vi "Main.vi"(8 "error in (no error)":errorcluster, 11 "AOTFBase in":refnum<class "AOTF.lvclass">) -> (0 "error out":errorcluster, 3 "component":refnum<class "AOTF.lvclass">)   [LabVIEW 2012, in "AOTF.lvclass"]
doc: "Main VI of the component."
uses:
  AOTF.lvclass
  <vilib>/Distrio/Murmex/Murmex/command_enum.ctl
  Controls/laser line ring.ctl
  <vilib>/Distrio/Murmex/InitialiseMessage/InitialiseMessage.lvclass
  AOTF.lvclass/AOTF.ctl
  <vilib>/Distrio/Murmex/ConfigureMessage/ConfigureMessage.lvclass
  <vilib>/Distrio/Murmex/TerminateMessage/TerminateMessage.lvclass
  <vilib>/Distrio/Murmex/Murmex/update_cluster.ctl
  <vilib>/Distrio/Murmex/Murmex/Set configure at initialise.vi
  <vilib>/Distrio/Murmex/Murmex/Set VI reference.vi
  <vilib>/Distrio/Murmex/Murmex/Get ID.vi
  <vilib>/Distrio/Murmex/Murmex/Set log reference.vi
  <vilib>/Distrio/Murmex/Murmex/Set write log to disk.vi
  <vilib>/Distrio/Murmex/Murmex/Murmex.lvclass
  <vilib>/Distrio/Murmex/Message/Message.lvclass
panel:
  in  "button::configure":bool
  in  "button::quit":bool
  out "terminate?":bool=TRUE
  in  "Tab Control":enum32{"Main", "Ramp", "Debug"}(tab)
  in  "Power":dbl(knob) caption="Power [%]" min=0.0 max=100.0 scale=0.0..100.0
  in  "Wavelength":T1=10 items=["Blind"=10, "405nm"=0, "445nm"=5, "491nm"=1, "515nm"=2, "561nm"=3]
  in  "Frame rate (Hz)":dbl
  in  "Number of frames":i32
  in  "Final power [%]":dbl
  in  "Start power [%]":dbl
  out "log":string="\r\n11:11:41.970 05/12/2013: initialise from AOTF to AOTF\r\n11:11:42.586 05/12/2013: inform from AOTF to AOTF\r\n11:11:43.913 05/12/2013: update from AOTF to AOTF\r\n11:11:45.142 05/12/2013: generic (shutter_off) from AOTF to AOTF\r\n11:11:45.270 05/12/2013: generic (shutter_on) from AOTF to AOTF\r\n11:11:45.902 05/12/2013: generic (shutter_off) from AOTF to AOTF\r\n11:11:45.932 05/12/2013: inspect from AOTF to AOTF\r\n11:11:48.013 05/12/2013: configure from AOTF to AOTF\r\n11:11:52.003 05/12/2013: inform from AOTF to AOTF\r\n11:11:58.521 05/12/2013: initialise from AOTF to AOTF\r\n11:11:58.561 05/12/2013: inform from AOTF to AOTF\r\n11:11:58.695 05/12/2013: inform from AOTF to AOTF\r\n11:12:02.089 05/12/2013: update from AOTF to AOTF\r\n11:12:02.308 05/12/2013: inspect from AOTF to AOTF\r\n11:12:02.364 05/12/2013: inform from AOTF to AOTF\r\n11:12:05.062 05/12/2013: generic (shutter_on) from AOTF to AOTF\r\n11:12:06.690 05/12/2013: update from AOTF to AOTF\r\n11:12:06.909 05/12/2013: inspect from AOTF to AOTF\r\n11:12:06.964 05/12/2013: inform from AOTF to AOTF\r\n11:12:07.770 05/12/2013: update from AOTF to AOTF\r\n11:12:07.989 05/12/2013: inspect from AOTF to AOTF\r\n11:12:08.044 05/12/2013: inform from AOTF to AOTF\r\n11:12:08.627 05/12/2013: update from AOTF to AOTF\r\n11:12:08.846 05/12/2013: inspect from AOTF to AOTF\r\n11:12:08.900 05/12/2013: inform from AOTF to AOTF\r\n11:12:09.290 05/12/2013: update from AOTF to AOTF\r\n11:12:09.508 05/12/2013: inspect from AOTF to AOTF\r\n11:12:09.563 05/12/2013: inform from AOTF to AOTF\r\n11:12:10.154 05/12/2013: update from AOTF to AOTF\r\n11:12:10.373 05/12/2013: inspect from AOTF to AOTF\r\n11:12:10.430 05/12/2013: inform from AOTF to AOTF\r\n11:12:20.953 05/12/2013: update from AOTF to AOTF\r\n11:12:21.172 05/12/2013: inspect from AOTF to AOTF\r\n11:12:21.227 05/12/2013: inform from AOTF to AOTF\r\n11:12:22.057 05/12/2013: update from AOTF to AOTF\r\n11:12:22.276 05/12/2013: inspect from AOTF to AOTF\r\n11:12:22.330 05/12/2013: inform from AOTF to AOTF\r\n11:12:22.841 05/12/2013: update from AOTF to AOTF\r\n11:12:23.060 05/12/2013: inspect from AOTF to AOTF\r\n11:12:23.114 05/12/2013: inform from AOTF to AOTF\r\n11:12:23.449 05/12/2013: update from AOTF to AOTF\r\n11:12:23.668 05/12/2013: inspect from AOTF to AOTF\r\n11:12:23.724 05/12/2013: inform from AOTF to AOTF\r\n11:12:24.514 05/12/2013: update from AOTF to AOTF\r\n11:12:24.733 05/12/2013: inspect from AOTF to AOTF\r\n11:12:24.789 05/12/2013: inform from AOTF to AOTF\r\n11:12:25.098 05/12/2013: update from AOTF to AOTF\r\n11:12:25.317 05/12/2013: inspect from AOTF to AOTF\r\n11:12:25.371 05/12/2013: inform from AOTF to AOTF\r\n11:12:26.482 05/12/2013: update from AOTF to AOTF\r\n11:12:26.701 05/12/2013: inspect from AOTF to AOTF\r\n11:12:26.755 05/12/2013: inform from AOTF to AOTF\r\n11:12:27.154 05/12/2013: update from AOTF to AOTF\r\n11:12:27.373 05/12/2013: inspect from AOTF to AOTF\r\n11:12:27.428 05/12/2013: inform from AOTF to AOTF\r\n11:12:27.666 05/12/2013: update from AOTF to AOTF\r\n11:12:27.885 05/12/2013: inspect from AOTF to AOTF\r\n11:12:27.944 05/12/2013: inform from AOTF to AOTF\r\n11:12:33.380 05/12/2013: update from AOTF to AOTF\r\n11:12:33.484 05/12/2013: update from AOTF to AOTF\r\n11:12:33.603 05/12/2013: inspect from AOTF to AOTF\r\n11:12:33.611 05/12/2013: update from AOTF to AOTF\r\n11:12:33.684 05/12/2013: update from AOTF to AOTF\r\n11:12:33.740 05/12/2013: update from AOTF to AOTF\r\n11:12:33.827 05/12/2013: inspect from AOTF to AOTF\r\n11:12:33.835 05/12/2013: update from AOTF to AOTF\r\n11:12:33.897 05/12/2013: inform from AOTF to AOTF\r\n11:12:33.903 05/12/2013: update from AOTF to AOTF\r\n11:12:33.940 05/12/2013: update from AOTF to AOTF\r\n11:12:34.085 05/12/2013: update from AOTF to AOTF\r\n11:12:34.119 05/12/2013: inspect from AOTF to AOTF\r\n11:12:34.292 05/12/2013: update from AOTF to AOTF\r\n11:12:34.336 05/12/2013: inspect from AOTF to AOTF\r\n11:12:34.553 05/12/2013: inspect from AOTF to AOTF\r\n11:12:34.608 05/12/2013: inform from AOTF to AOTF\r\n11:12:34.739 05/12/2013: update from AOTF to AOTF\r\n11:12:34.771 05/12/2013: update from AOTF to AOTF\r\n11:12:34.826 05/12/2013: inspect from AOTF to AOTF\r\n11:12:34.834 05/12/2013: update from AOTF to AOTF\r\n11:12:34.867 05/12/2013: update from AOTF to AOTF\r\n11:12:34.931 05/12/2013: update from AOTF to AOTF\r\n11:12:34.979 05/12/2013: update from AOTF to AOTF\r\n11:12:35.003 05/12/2013: update from AOTF to AOTF\r\n11:12:35.027 05/12/2013: update from AOTF to AOTF\r\n11:12:35.041 05/12/2013: update from AOTF to AOTF\r\n11:12:35.051 05/12/2013: inspect from AOTF to AOTF\r\n11:12:35.066 05/12/2013: update from AOTF to AOTF\r\n11:12:35.116 05/12/2013: update from AOTF to AOTF\r\n11:12:35.171 05/12/2013: update from AOTF to AOTF\r\n11:12:35.211 05/12/2013: update from AOTF to AOTF\r\n11:12:35.273 05/12/2013: inspect from AOTF to AOTF\r\n11:12:35.287 05/12/2013: update from AOTF to AOTF\r\n11:12:35.475 05/12/2013: update from AOTF to AOTF\r\n11:12:35.495 05/12/2013: inspect from AOTF to AOTF\r\n11:12:35.549 05/12/2013: inform from AOTF to AOTF\r\n11:12:35.764 05/12/2013: inspect from AOTF to AOTF\r\n11:12:35.819 05/12/2013: inform from AOTF to AOTF\r\n11:12:35.861 05/12/2013: update from AOTF to AOTF\r\n11:12:35.877 05/12/2013: inform from AOTF to AOTF\r\n11:12:35.947 05/12/2013: update from AOTF to AOTF\r\n11:12:36.067 05/12/2013: update from AOTF to AOTF\r\n11:12:36.100 05/12/2013: inspect from AOTF to AOTF\r\n11:12:36.235 05/12/2013: update from AOTF to AOTF\r\n11:12:36.317 05/12/2013: inspect from AOTF to AOTF\r\n11:12:36.371 05/12/2013: inform from AOTF to AOTF\r\n11:12:36.587 05/12/2013: inspect from AOTF to AOTF\r\n11:12:36.771 05/12/2013: update from AOTF to AOTF\r\n11:12:36.804 05/12/2013: inspect from AOTF to AOTF\r\n11:12:37.020 05/12/2013: inspect from AOTF to AOTF\r\n11:12:37.238 05/12/2013: inspect from AOTF to AOTF\r\n11:12:37.456 05/12/2013: inspect from AOTF to AOTF\r\n11:12:37.673 05/12/2013: inspect from AOTF to AOTF\r\n11:12:37.891 05/12/2013: inspect from AOTF to AOTF\r\n11:12:37.946 05/12/2013: inform from AOTF to AOTF\r\n11:12:38.161 05/12/2013: inspect from AOTF to AOTF\r\n11:12:38.379 05/12/2013: inspect from AOTF to AOTF\r\n11:12:38.597 05/12/2013: inspect from AOTF to AOTF\r\n11:12:38.815 05/12/2013: inspect from AOTF to AOTF\r\n11:12:38.871 05/12/2013: inform from AOTF to AOTF\r\n11:12:39.086 05/12/2013: inspect from AOTF to AOTF\r\n11:12:39.303 05/12/2013: inspect from AOTF to AOTF\r\n11:12:39.363 05/12/2013: inform from AOTF to AOTF\r\n11:12:39.417 05/12/2013: inform from AOTF to AOTF\r\n11:12:39.633 05/12/2013: inspect from AOTF to AOTF\r\n11:12:39.852 05/12/2013: inspect from AOTF to AOTF\r\n11:12:40.069 05/12/2013: inspect from AOTF to AOTF\r\n11:12:40.124 05/12/2013: inform from AOTF to AOTF\r\n11:12:40.339 05/12/2013: inspect from AOTF to AOTF\r\n11:12:40.395 05/12/2013: inform from AOTF to AOTF\r\n11:12:40.448 05/12/2013: inform from AOTF to AOTF\r\n11:12:40.663 05/12/2013: inspect from AOTF to AOTF\r\n11:12:40.718 05/12/2013: inform from AOTF to AOTF\r\n11:12:40.770 05/12/2013: inform from AOTF to AOTF\r\n11:12:40.824 05/12/2013: inform from AOTF to AOTF\r\n11:12:40.877 05/12/2013: inform from AOTF to AOTF\r\n11:12:40.930 05/12/2013: inform from AOTF to AOTF\r\n11:12:40.982 05/12/2013: inform from AOTF to AOTF\r\n11:12:41.034 05/12/2013: inform from AOTF to AOTF\r\n11:12:41.092 05/12/2013: inform from AOTF to AOTF\r\n11:12:41.144 05/12/2013: inform from AOTF to AOTF\r\n11:12:41.196 05/12/2013: inform from AOTF to AOTF\r\n11:12:41.249 05/12/2013: inform from AOTF to AOTF\r\n11:12:41.307 05/12/2013: inform from AOTF to AOTF\r\n11:12:41.366 05/12/2013: inform from AOTF to AOTF\r\n11:12:41.424 05/12/2013: inform from AOTF to AOTF\r\n11:12:41.478 05/12/2013: inform from AOTF to AOTF\r\n11:12:41.533 05/12/2013: inform from AOTF to AOTF\r\n11:12:41.589 05/12/2013: inform from AOTF to AOTF\r\n11:12:42.246 05/12/2013: terminate from AOTF to AOTF"
  in  "component ID":string="AOTF"
  in  "button::send":bool
  in  "command":T2
  in  "Generic command":string
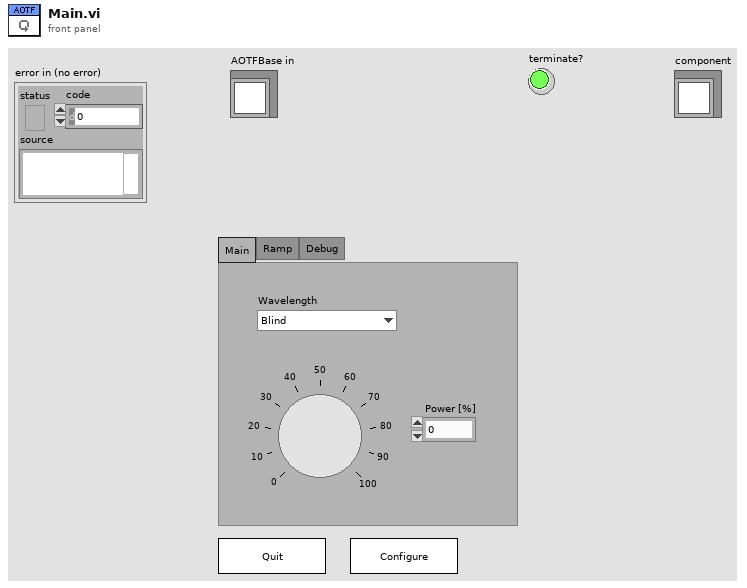
[diagram p1: front panel]
types:
  T1 = typedef "AOTF.lvclass/laser line ring.ctl" = u8
  T2 = typedef "Murmex.lvlib/Murmex.lvclass/command_enum.ctl" = enum16{"null", "initialise", "reset", "terminate", "acknowledge", "update", "inspect", "inform", "proceed", "start", "stop", "fetch", "configure", "generic"}
  T3 = enum8{"Enabled", "Disabled", "Disabled and Grayed Out"}
  T4 = typedef "Murmex.lvlib/Murmex.lvclass/update_cluster.ctl" = cluster{"target ID":string, "key chains":string[], "values":variant[]}
  T5 = typedef "Murmex.lvclass/command_enum.ctl" = enum16{"null", "initialise", "reset", "terminate", "acknowledge", "update", "inspect", "inform", "proceed", "start", "stop", "fetch", "configure", "generic"}
  T6 = typedef "Murmex.lvclass/Event type enumerations.ctl" = enum16{"before", "after"}
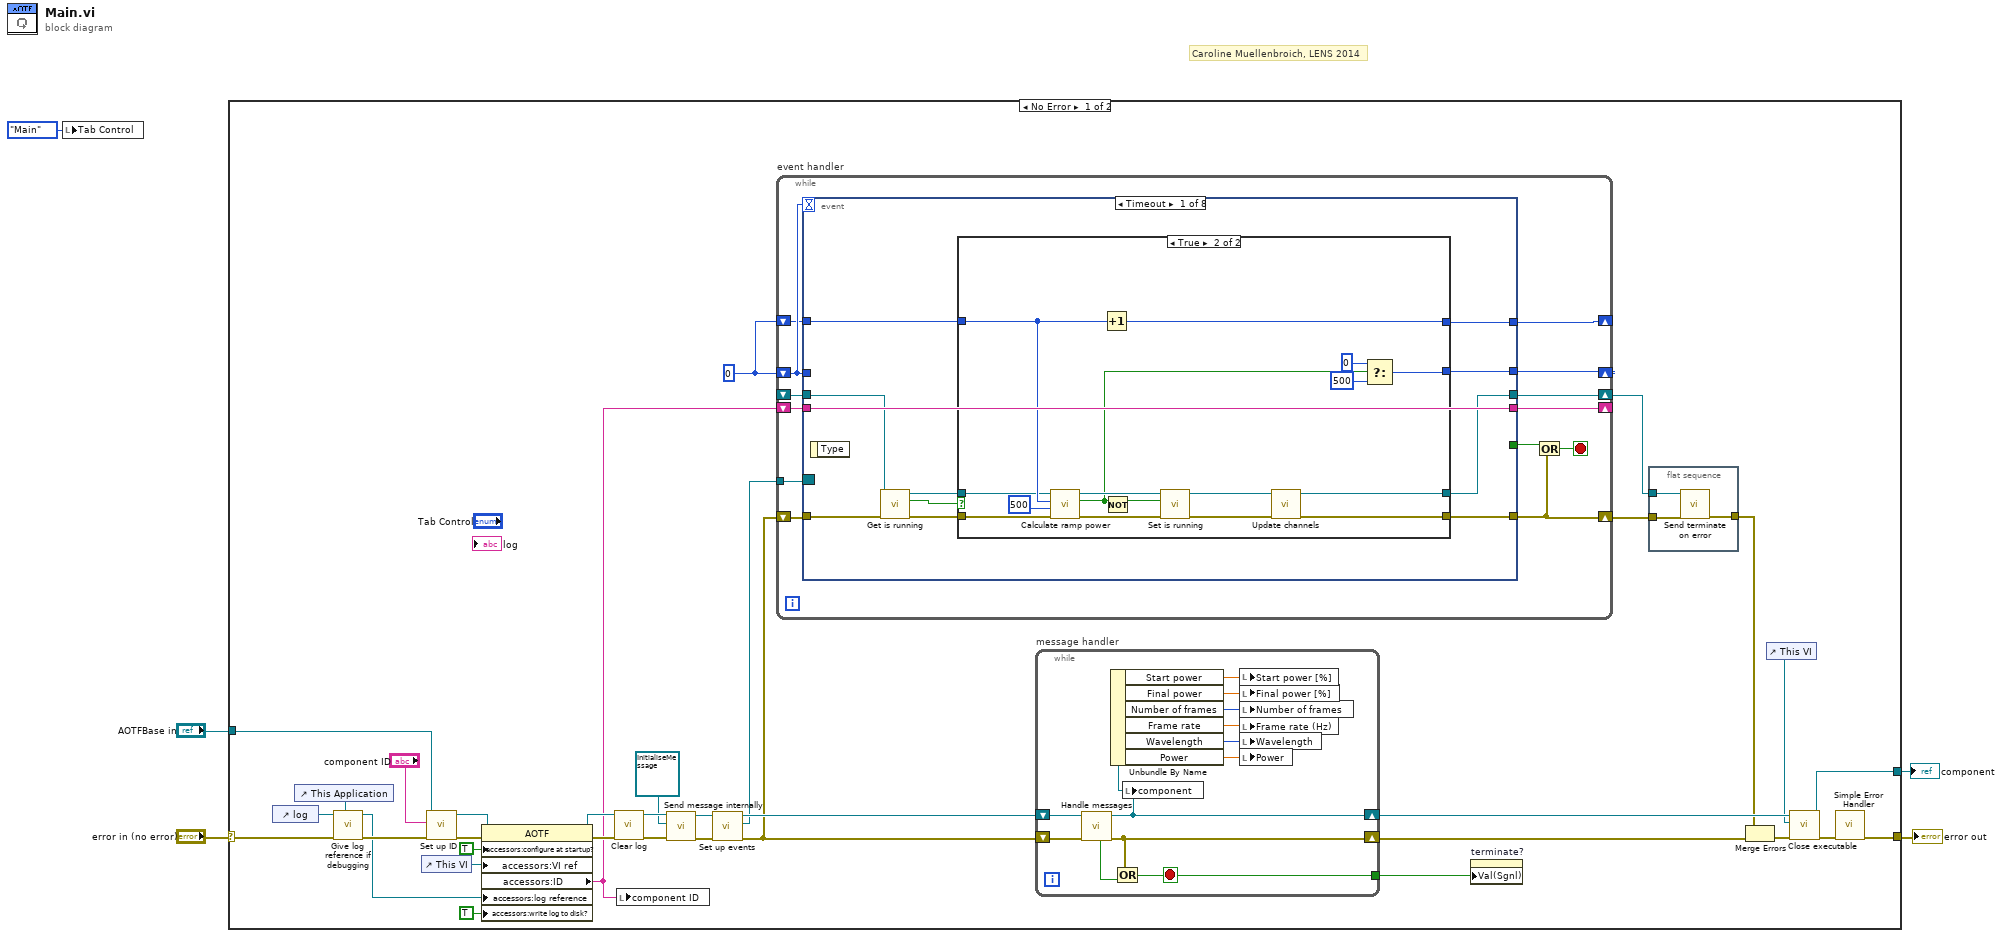
[diagram p0: block diagram]
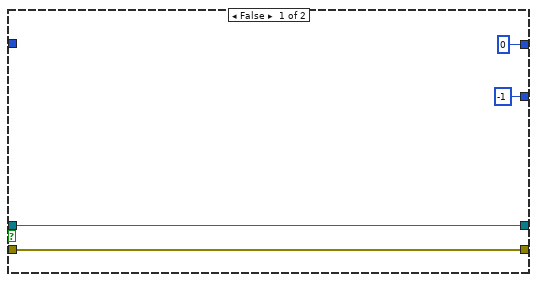
[diagram p2: hidden frame]
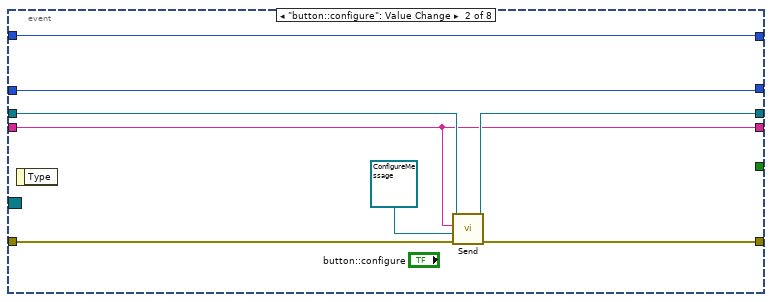
[diagram p3: hidden frame]
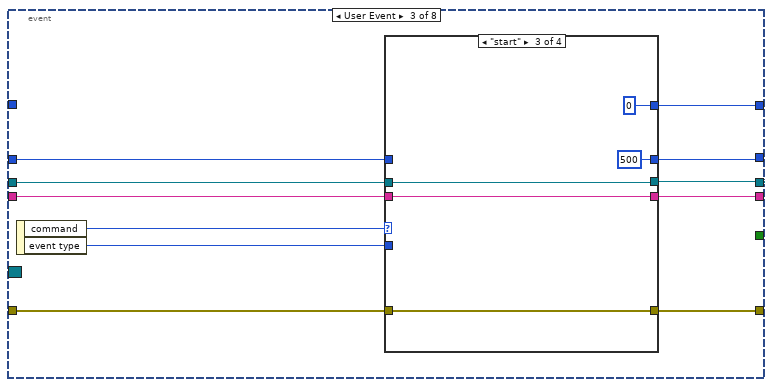
[diagram p4: hidden frame]
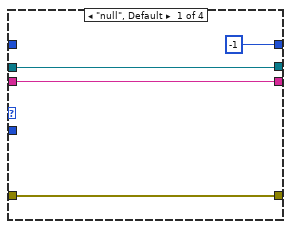
[diagram p5: hidden frame]
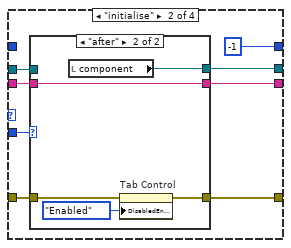
[diagram p6: hidden frame]
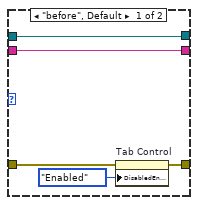
[diagram p7: hidden frame]
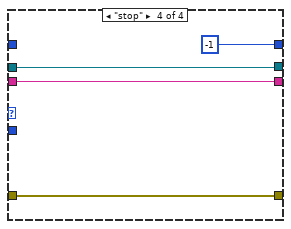
[diagram p8: hidden frame]
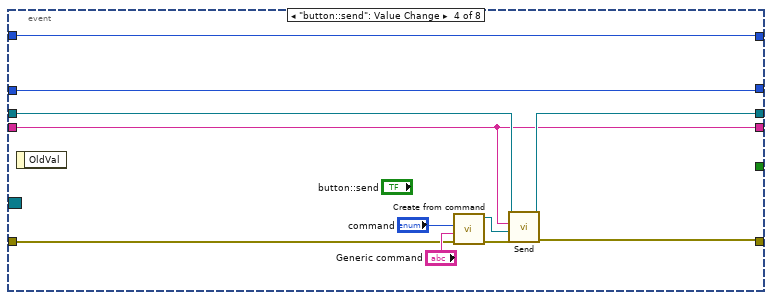
[diagram p9: hidden frame]
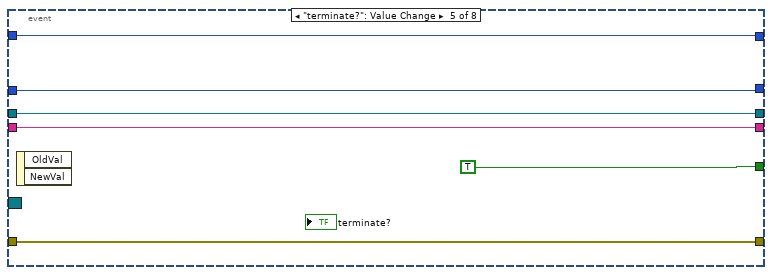
[diagram p10: hidden frame]
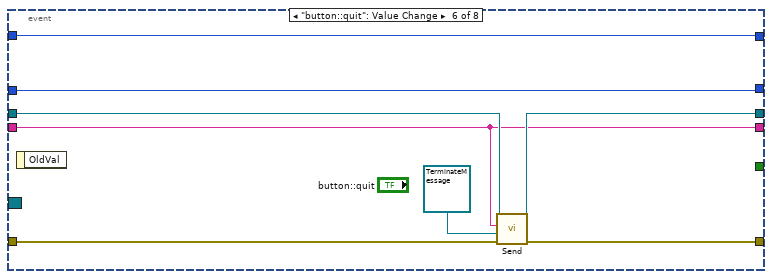
[diagram p11: hidden frame]
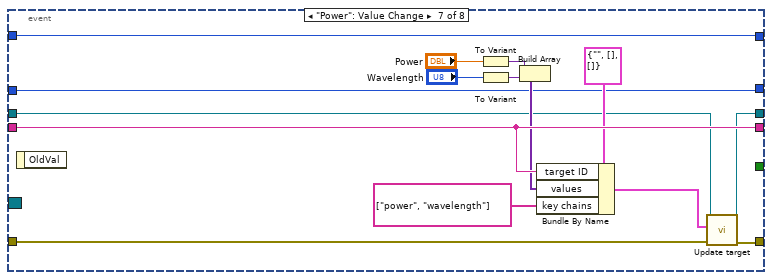
[diagram p12: hidden frame]
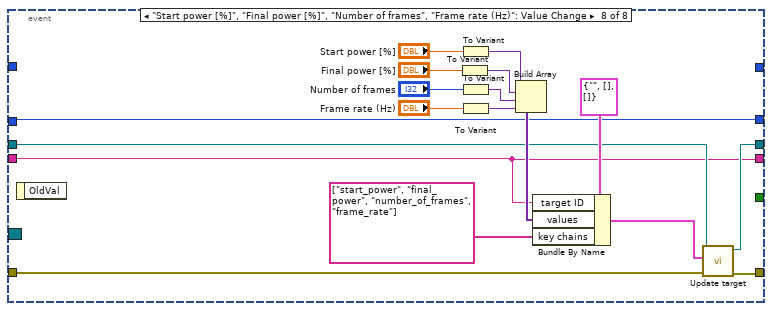
[diagram p13: hidden frame]
diagram:
  # "Caroline Muellenbroich, LENS 2014"
  n1 = local write "Tab Control"(enum32{"Main", "Ramp", "Debug"}."Main" ("Tab Control")) -> ()
  n2 = case shown="No Error" "error in (no error)" {
    selector: "error in (no error)" -> [w11 w209]
    tunnel: "AOTFBase in" -> [w40 w208]
    tunnel: [w25 w208] -> w5
    tunnel: [w21 w209] -> w4
    frame No Error {
      w6 = 0
      n3 = control-ref of="log"() -> (w12:refnum<vi>)
      n4 = control-ref of="This Application"() -> (w13:refnum<vi>)
      n5 = call "Give log reference if debugging.vi"("application ref"=w13, "error in (no error)"=w11, "log reference in"=w12) -> ("error out"=w10:errorcluster, "log reference out"=w9:refnum<vi>)  [unwired: 6 in, 1 out]
      n6 = control-ref of="This VI"() -> (w36:refnum<vi>)
      n7 = call <vilib>:"Set up ID.vi"("error in (no error)"=w10, "component ID"="component ID", "MurmexBase in"=w40) -> ("error out"=w39:errorcluster, "MurmexBase out"=w38:refnum<class "AOTF.lvclass">)  [unwired: 6 in, 1 out]
      n8 = property class="AOTF"(reference=w38, error in=w39, "accessors:configure at startup?"=TRUE ("configure at startup?"), "accessors:VI ref"=w36, "accessors:log reference"=w9, "accessors:write log to disk?"=TRUE ("write log to disk?")) -> (reference out=w33:refnum<class "AOTF.lvclass">, error out=w35:errorcluster, "accessors:ID"=w16:string)
      n9 = call <vilib>:"Clear log.vi"("error in (no error)"=w35, "MurmexBase in"=w33) -> ("error out"=w34:errorcluster, "MurmexBase out"=w32:refnum<class "AOTF.lvclass">)  [unwired: 8 in]
      n10 = local write "component ID"(w16) -> ()
      n11 = call <vilib>:"Send message internally.vi"("error in (no error)"=w34, "Message"=refnum<class "InitialiseMessage.lvclass"> refnum ("Murmex.lvlib:InitialiseMessage"), "Murmex in"=w32) -> ("error out"=w31:errorcluster, "Murmex out"=w8:refnum<class "AOTF.lvclass">)  [unwired: 7 in]
      n12 = call <vilib>:"Set up events.vi"("error in (no error)"=w31, "MurmexBase in"=w8) -> ("error out"=w24:errorcluster, "Event Registration Refnum"=w23:refnum<event-registration>, "MurmexBase out"=w30:refnum<class "AOTF.lvclass">)  [unwired: 7 in]
      n13 = while "event handler" {
        tunnel: w23 -> [w56]
        shift-right: [w49] -> w20
        shift-left: w24 -> [w55]
        shift-right: [w51] -> _
        shift-left: w16 -> [w54]
        shift-right: [w53] -> w18
        shift-left: _ -> [w52]
        shift-right: [w47] -> _
        shift-left: w6 -> [w46]
        shift-right: [w45] -> _
        shift-left: w6 -> [w44]
        stop <- w50 stop-if-true
        n14 = event shown="[0] Timeout" {
          selector: w56 -> [_ _ _ _ _ _ _ _]
          dyn-events: _ -> [_ _ _ _ _ _ _ _]
          timeout: w46 -> [_ _ _ _ _ _ _ _]
          tunnel: w55 -> [w66 w95 w104 w145 w154 w162 w176 w190]
          tunnel: [w61 w94 w103 w144 w154 w161 w177 w189] -> w49
          tunnel: w54 -> [w67 w90 w102 w140 w152 w157 w175 w185]
          tunnel: [w59 w92 w101 w142 w151 w159 w170 w188] -> w53
          tunnel: w52 -> [w65 w93 w100 w143 w151 w160 w166 w187]
          tunnel: [w67 w90 w99 w140 w152 w157 w175 w185] -> w51
          tunnel: [_ _ _ _ TRUE _ _ _] -> w48
          tunnel: w46 -> [_ w91 w97 w141 w150 w158 w167 w186]
          tunnel: [w64 w91 w98 w141 w150 w158 w167 w186] -> w47
          tunnel: [w62 w88 w96 w138 w149 w155 w163 _] -> w45
          tunnel: w44 -> [w57 w88 _ w138 w149 w155 w163 _]
          event Timeout {
            n15 = event-data() -> ()  [unwired: 1 in, 1 out]
            n16 = call-dynamic "Get is running.vi"("error in (no error)"=w66, "AOTF in"=w65) -> ("error out"=w60:errorcluster, "is running?"=w63:bool, "AOTF out"=w58:refnum<class "AOTF.lvclass">)  [unwired: 7 in]
            n17 = case shown="True" w63 {
              tunnel: [-1 ("t") w72] -> w64
              tunnel: [0 ("t") w87] -> w62
              tunnel: [w69 w80] -> w61
              tunnel: w60 -> [w69 w84]
              tunnel: [w68 w81] -> w59
              tunnel: w58 -> [w68 w83]
              tunnel: w57 -> [_ w85]
              frame False {
              }
              frame True {
                n18 = call-dynamic "Calculate ramp power.vi"("error in (no error)"=w84, "Time between updates (ms)"=500 ("t"), "Current update"=w85, "AOTF in"=w83) -> ("error out"=w82:errorcluster, "finished?"=w74:bool, "AOTF out"=w78:refnum<class "AOTF.lvclass">)  [unwired: 5 in]
                n19 = Increment(x=w85) -> (x+1=w87:i32)
                n20 = Not(x=w74) -> (.not. x?=w76:bool)
                n21 = call-dynamic "Set is running.vi"("error in (no error)"=w82, "is running?"=w76, "AOTF in"=w78) -> ("error out"=w79:errorcluster, "AOTF out"=w77:refnum<class "AOTF.lvclass">)  [unwired: 7 in]
                n22 = call-dynamic "Update channels.vi"("error in (no error)"=w79, "AOTF in"=w77) -> ("error out"=w80:errorcluster, "AOTF out"=w81:refnum<class "AOTF.lvclass">)  [unwired: 8 in]
                n23 = Select(t=0, s=w74, f=500 ("t")) -> (s? t:f=w72:i32)
              }
            }
          }
          event "button::configure": Value Change {
            n24 = event-data() -> ()  [unwired: 1 in, 1 out]
            n25 = call <vilib>:"Send.vi"("error in (no error)"=w95, "Message"=refnum<class "ConfigureMessage.lvclass"> refnum ("Murmex.lvlib:ConfigureMessage"), "recipient"=w90, "Murmex in"=w93) -> ("error out"=w94:errorcluster, "Murmex out"=w92:refnum<class "AOTF.lvclass">)  [unwired: 6 in]
          }
          event User Event {
            n26 = event-data() -> ("command"=w106:T5, "event type"=w105:T6)  [unwired: 1 in]
            n27 = case shown="\"start\"" w106 {
              tunnel: w105 -> [_ w118 _ _]
              tunnel: w104 -> [w108 w117 w131 w135]
              tunnel: [w108 w116 w131 w135] -> w103
              tunnel: w102 -> [w110 w115 w132 w136]
              tunnel: [w109 w114 w133 w137] -> w101
              tunnel: w100 -> [w109 w113 w133 w137]
              tunnel: [w110 w112 w132 w136] -> w99
              tunnel: [-1 -1 500 -1] -> w98
              tunnel: w97 -> [_ _ _ _]
              tunnel: [_ _ 0 _] -> w96
              frame "null", Default {
              }
              frame "initialise" {
                n28 = case shown="\"after\"" w118 {
                  tunnel: [w122 w127] -> w116
                  tunnel: w117 -> [w123 w128]
                  tunnel: w115 -> [w120 w125]
                  tunnel: [w119 w124] -> w114
                  tunnel: w113 -> [w119 _]
                  tunnel: [w120 w125] -> w112
                  frame "before", Default {
                    n29 = property on="Tab Control" class="TabCtl (strict)"(error in=w123, "DisabledEnum"=T3."Enabled" ("Disabled")) -> (error out=w122:errorcluster)  [unwired: 1 in, 1 out]
                  }
                  frame "after" {
                    n30 = local read "component"() -> (w124:refnum<class "AOTF.lvclass">)
                    n31 = property on="Tab Control" class="TabCtl (strict)"(error in=w128, "DisabledEnum"=T3."Enabled" ("Disabled")) -> (error out=w127:errorcluster)  [unwired: 1 in, 1 out]
                  }
                }
              }
              frame "start" {
              }
              frame "stop" {
              }
            }
          }
          event "button::send": Value Change {
            n32 = event-data() -> ()  [unwired: 1 in, 1 out]
            n33 = call <vilib>:"Create from command.vi"("error in (no error)"=w145, "generic command"="Generic command", "command"="command") -> ("error out"=w147:errorcluster, "Message out"=w146:refnum<class "Message.lvclass">)  [unwired: 7 in]
            n34 = call <vilib>:"Send.vi"("error in (no error)"=w147, "Message"=w146, "recipient"=w140, "Murmex in"=w143) -> ("error out"=w144:errorcluster, "Murmex out"=w142:refnum<class "AOTF.lvclass">)  [unwired: 6 in]
          }
          event "terminate?": Value Change {
            n35 = event-data() -> ()  [unwired: 1 in, 2 out]
          }
          event "button::quit": Value Change {
            n36 = event-data() -> ()  [unwired: 1 in, 1 out]
            n37 = call <vilib>:"Send.vi"("error in (no error)"=w162, "Message"=refnum<class "TerminateMessage.lvclass"> refnum ("Murmex.lvlib:TerminateMessage"), "recipient"=w157, "Murmex in"=w160) -> ("error out"=w161:errorcluster, "Murmex out"=w159:refnum<class "AOTF.lvclass">)  [unwired: 6 in]
          }
          event "Power": Value Change {
            n38 = event-data() -> ()  [unwired: 1 in, 1 out]
            n39 = To Variant(anything="Power") -> (Variant=w169:variant)
            n40 = To Variant(anything="Wavelength") -> (Variant=w168:variant)
            n41 = Build Array(w169, w168) -> (w171:variant[])
            n42 = Bundle By Name(cluster=T4 {"target ID"="", "key chains"=[], "values"=[]} ("update cluster"), "target ID"=w175, "values"=w171, "key chains"=string[] ["power", "wavelength"]) -> (w174:T4)
            n43 = call <vilib>:"Update target.vi"("error in (no error)"=w176, "update cluster"=w174, "MurmexBase in"=w166) -> ("error out"=w177:errorcluster, "MurmexBase out"=w170:refnum<class "AOTF.lvclass">)  [unwired: 7 in]
          }
          event "Start power [%]", "Final power [%]", "Number of frames", "Frame rate (Hz)": Value Change {
            n44 = event-data() -> ()  [unwired: 1 in, 1 out]
            n45 = To Variant(anything="Final power [%]") -> (Variant=w183:variant)
            n46 = To Variant(anything="Start power [%]") -> (Variant=w182:variant)
            n47 = To Variant(anything="Number of frames") -> (Variant=w184:variant)
            n48 = To Variant(anything="Frame rate (Hz)") -> (Variant=w191:variant)
            n49 = Build Array(w182, w183, w184, w191) -> (w192:variant[])
            n50 = Bundle By Name(cluster=T4 {"target ID"="", "key chains"=[], "values"=[]} ("update cluster"), "target ID"=w185, "values"=w192, "key chains"=string[] ["start_power", "final_power", "number_of_frames", "frame_rate"]) -> (w195:T4)
            n51 = call <vilib>:"Update target.vi"("error in (no error)"=w190, "update cluster"=w195, "MurmexBase in"=w187) -> ("error out"=w189:errorcluster, "MurmexBase out"=w188:refnum<class "AOTF.lvclass">)  [unwired: 7 in]
          }
        }
        n52 = Or(x=w48, y=w49) -> (x .or. y?=w50:bool)
      }
      n53 = while "message handler" {
        shift-right: [w202] -> w26
        shift-left: w30 -> [w206]
        shift-right: [w205] -> w27
        shift-left: w24 -> [w207]
        tunnel: [w203] -> w22
        stop <- w203 stop-if-true
        n54 = call <vilib>:"Handle messages.vi"("error in (no error)"=w207, "Murmex in"=w206) -> ("error out"=w205:errorcluster, "Murmex out"=w202:refnum<class "AOTF.lvclass">, "terminated?"=w204:bool)  [unwired: 7 in]
        n55 = Unbundle By Name(w202) -> ("Start power"=w199:dbl, "Final power"=w198:dbl, "Number of frames"=w197:i32, "Frame rate"=w196:dbl, "Wavelength"=w200:T1, "Power"=w201:dbl)
        n56 = Or(x=w205, y=w204) -> (x .or. y?=w203:bool)
        n57 = local write "component"(w202) -> ()
        n58 = local write "Start power [%]"(w199) -> ()
        n59 = local write "Final power [%]"(w198) -> ()
        n60 = local write "Number of frames"(w197) -> ()
        n61 = local write "Frame rate (Hz)"(w196) -> ()
        n62 = local write "Wavelength"(w200) -> ()
        n63 = local write "Power"(w201) -> ()
      }
      n64 = property on="terminate?" class="Bool (strict)"("Val(Sgnl)"=w22) -> ()  [unwired: 2 in, 2 out]
      n65 = flat-sequence {
        tunnel: w20 -> [w42]
        tunnel: [w43] -> w19
        tunnel: w18 -> [w41]
        frame #0 {
          n66 = call <vilib>:"Send terminate on error.vi"("error in (no error)"=w42, "Murmex in"=w41) -> ("error out"=w43:errorcluster)  [unwired: 8 in, 1 out]
        }
      }
      n67 = Merge Errors(w19, w27) -> (w28:errorcluster)
      n68 = control-ref of="This VI"() -> (w17:refnum<vi>)
      n69 = call <vilib>:"Close executable.vi"("error in (no error)"=w28, "main VI ref (optional)"=w17, "MurmexBase in"=w26) -> ("error out"=w29:errorcluster, "MurmexBase out"=w25:refnum<class "AOTF.lvclass">)  [unwired: 7 in]
      n70 = call <vilib>:"Simple Error Handler.vi"("error in (no error)"=w29) -> ("error out"=w21:errorcluster)  [unwired: 4 in, 4 out]
    }
    frame Error {
    }
  }
  "error out" <- w4
  "component" <- w5
